vi "Initialize AO Channels.vi"(8 "error in (no error)":errorcluster, 11 "Instrument.DAQ":refnum<class "Instrument.DAQ.lvclass">) -> (0 "error out":errorcluster, 3 "Instrument.DAQ out":refnum<class "Instrument.DAQ.lvclass">)   [LabVIEW 2019, in "Instrument.DAQ.lvclass"]
uses:
  Instrument.DAQ.lvclass
  Instrument.DAQ.lvclass/Instrument.DAQ.ctl
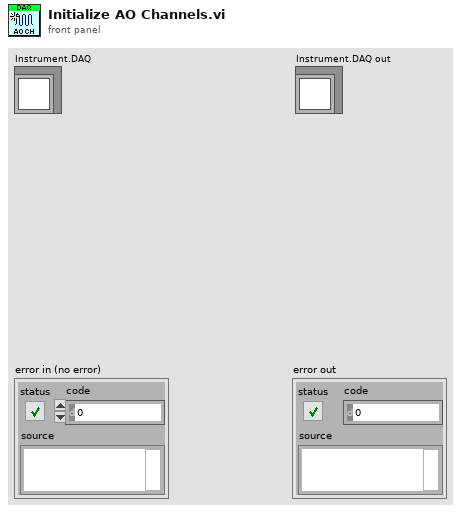
[diagram p1: front panel]
types:
  T1 = typedef "Instrument.DAQ.lvclass/AO.Channel--Cluster--Array.ctl" = T2[]
  T2 = typedef "Instrument.DAQ.lvclass/AO.Channel--Cluster.ctl" = cluster{"Enable?":bool, "Channel":i32, "Amplitude":dbl, "Offset":dbl, "Frequency":dbl, "Phase":dbl, "Function":T3, "Sweeping?":bool}
  T3 = typedef "Instrument.DAQ.lvclass/AO.Channel.Function--Enum.ctl" = enum16{"Sine", "Triangle", "Square"}
  T4 = typedef "Instrument.DAQ.lvclass/DAQ.Config.AO--Cluster--Array.ctl" = T5[]
  T5 = typedef "Instrument.DAQ.lvclass/DAQ.Config.AO--Cluster.ctl" = cluster{"Channels":tag, "Range":T6, "output terminal configuration":i32, "Type":T7}
  T6 = typedef "Instrument.DAQ.lvclass/DAQ.Config.AO.Range--enum.ctl" = enum16{"±0.1", "±1.0", "±10.0"}
  T7 = typedef "Instrument.DAQ.lvclass/DAQ.Type--enum.ctl" = enum16{"None", "USB 4431", "PXI 446x"}
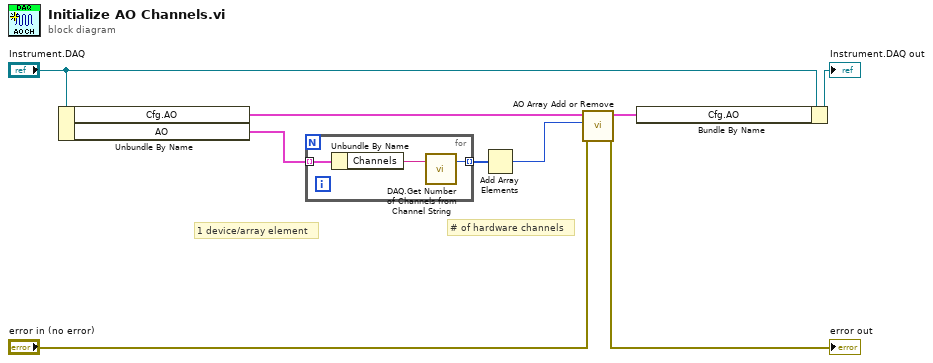
[diagram p0: block diagram]
diagram:
  # "1 device/array element"
  # "# of hardware channels"
  n1 = Unbundle By Name("Instrument.DAQ") -> ("Cfg.AO"=w2:T1, "AO"=w1:T4)
  n2 = for {
    tunnel: w1 -> [w12] mode=indexing
    tunnel: [w11] -> w9 mode=indexing
    n3 = Unbundle By Name(w12) -> ("Channels"=w10:tag)
    n4 = call "DAQ.Get Number of Channels from Channel String.vi"("Channels String"=w10) -> ("# channels"=w11:i32)  [unwired: 2 in]
  }
  n5 = Add Array Elements(numeric array=w9) -> (sum=w5:i32)
  n6 = call "AO Array Add or Remove.vi"("error in (no error)"="error in (no error)", "Size"=w5, "AO Channels in"=w2) -> ("error out"=→"error out":errorcluster, "AO Channels out"=w6:T1)  [unwired: 7 in]
  n7 = Bundle By Name(cluster="Instrument.DAQ", "Cfg.AO"=w6) -> (→"Instrument.DAQ out":refnum<class "Instrument.DAQ.lvclass">)
